vi "DockGUI.vi"(8 "ErrorIn":errorcluster, 9 "SubPanelName":string, 10 "ObjectName":string, 11 "ObjectIn":refnum<class "IDockGUI.lvclass">) -> (0 "ErrorOut":errorcluster, 3 "ObjectOut":refnum<class "IDockGUI.lvclass">)   [LabVIEW 2021, in "IDockGUI.lvclass"]
uses:
  IDockGUI.lvclass
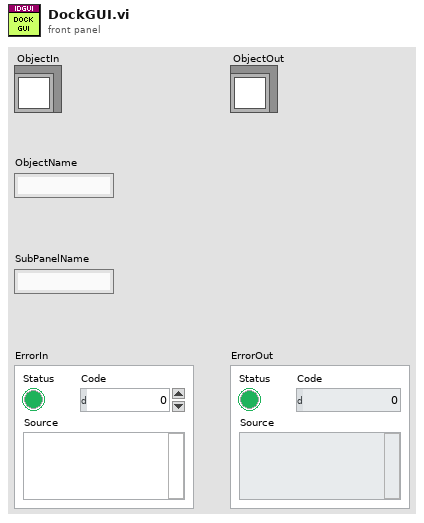
[diagram p1: front panel]
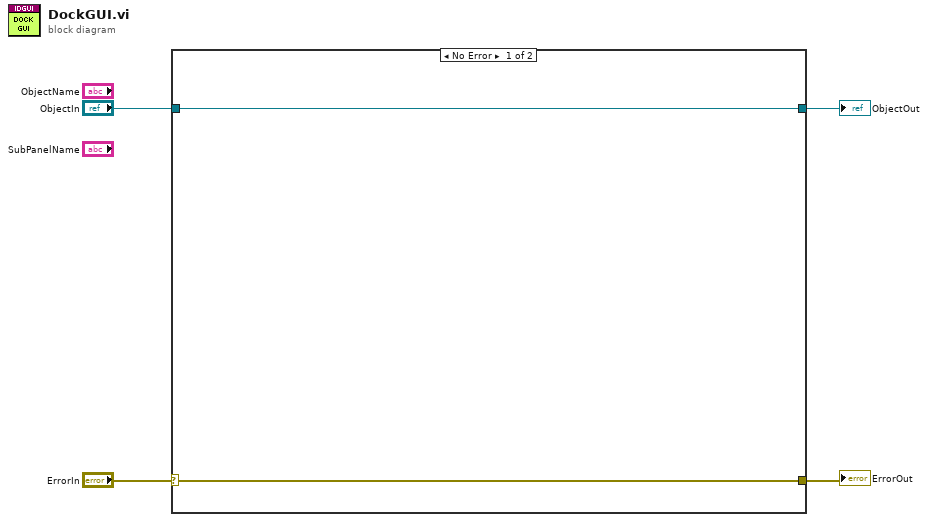
[diagram p0: block diagram]
diagram:
  n1 = case shown="No Error" "ErrorIn" {
    selector: "ErrorIn" -> [w6 w8]
    tunnel: [w6 w8] -> w3
    tunnel: [w5 w7] -> w1
    tunnel: "ObjectIn" -> [w5 w7]
    frame No Error {
    }
    frame Error {
    }
  }
  "ErrorOut" <- w3
  "ObjectOut" <- w1
